vi "qFPH.vi"(0 "System no.":i32=1 min=1 max=4 step=1, 2 "Axes to query":string[](array[string]), 3 "All axes?":bool, 4 "Axis identifier?":bool=TRUE, 5 "error in":errorcluster) -> (14 "Phase offset":dbl[](array[numeric]) format="%.6f", 19 "error out":errorcluster)   [LabVIEW 2026]
doc: "Returns phase offset for queried axes.\n\nAll systems: If All axes? = TRUE, then Axis identifier? can be FALSE"
panel:
  # "Returns phase offset of queried axes."
  # "If all axes: use"
  # "Query"
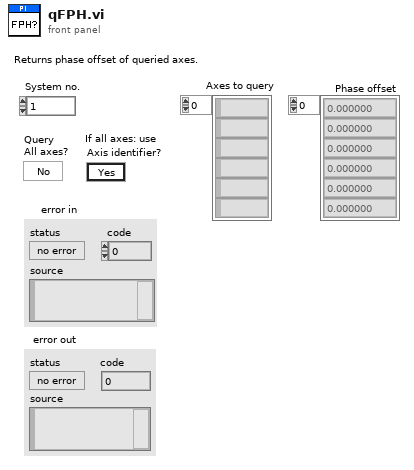
[diagram p1: front panel]
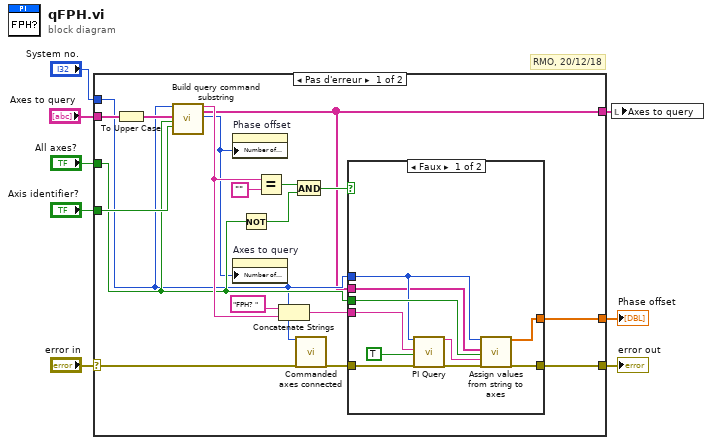
[diagram p0: block diagram]
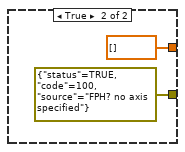
[diagram p2: hidden frame]
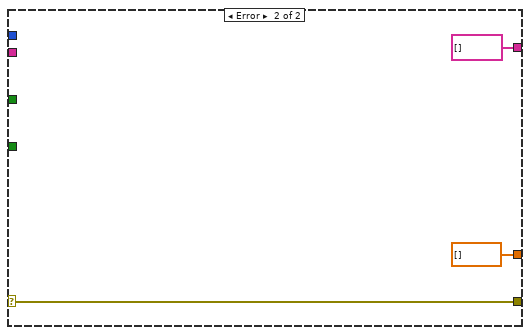
[diagram p3: hidden frame]
diagram:
  # "RMO, 20/12/18"
  n1 = case shown="Pas d'erreur" "error in" {
    selector: "error in" -> [w9 w39]
    tunnel: "Axes to query" -> [w24 _]
    tunnel: "Axis identifier?" -> [w21 _]
    tunnel: "All axes?" -> [w16 _]
    tunnel: [w17 dbl[] [] ("Values")] -> w5
    tunnel: [w13 w39] -> w4
    tunnel: "System no." -> [w12 _]
    tunnel: [w10 string[] [] ("Axes to query out")] -> w2
    frame No Error {
      n2 = To Upper Case(1:w24) -> (0:w22:string[])
      n3 = call "Build query command substring.vi"("System no."=w12, "Axes to query in"=w22, "Query\nAll axes?"=w16, "For all axes: use\nAxis identifier?"=w21) -> ("Command substring"=w20:string, "Axes to query out"=w10:string[], "Number of rows"=w15:u32)  [unwired: 2 in, 11 out]
      n4 = property on="Phase offset" class="Tabl (strict)"("Number of Rows"=w15) -> ()  [unwired: 2 in, 2 out]
      n5 = property on="Axes to query" class="Tabl (strict)"("Number of Rows"=w15) -> ()  [unwired: 2 in, 2 out]
      n6 = Not(x=w16) -> (.not. x?=w18:bool)
      n7 = Equal?(x=w20, y="" ("x")) -> (x = y?=w19:bool)
      n8 = Concatenate Strings("FPH? ", w20) -> (w25:string)
      n9 = And(x=w19, y=w18) -> (x .and. y?=w14:bool)
      n10 = call "Commanded axes connected.vi"("System no."=w12, "error in"=w9) -> ("error out"=w11:errorcluster)  [unwired: 2 in, 15 out]
      n11 = case shown="Faux" w14 {
        tunnel: w25 -> [w35 _]
        tunnel: [w34 dbl[] [] ("Values")] -> w17
        tunnel: w16 -> [w33 _]
        tunnel: [w32 errorcluster {"status"=TRUE, "code"=100, "source"="FPH? no axis specified"} ("error out")] -> w13
        tunnel: w12 -> [w31 _]
        tunnel: w11 -> [w30 _]
        tunnel: w10 -> [w29 _]
        frame False {
          n12 = call "PI Query.vi"("System no."=w31, "String to send"=w35, "Attach termination char.?"=TRUE ("Attach Linefeed?"), "error in"=w30) -> ("String read"=w27:string, "error out"=w28:errorcluster)  [unwired: 3 in, 11 out]
          n13 = call "Assign values from string to axes.vi"("System no."=w31, "Queried axes"=w29, "All axes queried?"=w33, "Input String"=w27, "error in"=w28) -> ("Values"=w34:dbl[], "error out"=w32:errorcluster)  [unwired: 1 in, 12 out]
        }
        frame True {
        }
      }
    }
    frame Error {
    }
  }
  "error out" <- w4
  "Phase offset" <- w5
  n14 = local write "Axes to query"(w2) -> ()
